vi "Fetch2ChSegHZOffset.vi"(9 "2nd Channel?":bool, 10 "Num Segs":i32=50, 11 "VISA resource name":refnum<visa-resource-name>="HDO6104") -> (0 "Run Time":u32, 1 "Array 2":dbl[](array[numeric]), 2 "Array":dbl[](array[numeric]), 3 "VISA resource name out":refnum<visa-resource-name>)   [LabVIEW 2022 SP3]
uses:
  <instrlib>/LeCroy Wave Series/LeCroy Wave Series.lvlib
panel:
  out "CH2 HZ Offset":dbl[](graph)
  out "CH1 HZ Offset":dbl[](graph)
  out "x-y":dbl[](array[numeric])
  out "Offset differences":dbl[](graph)
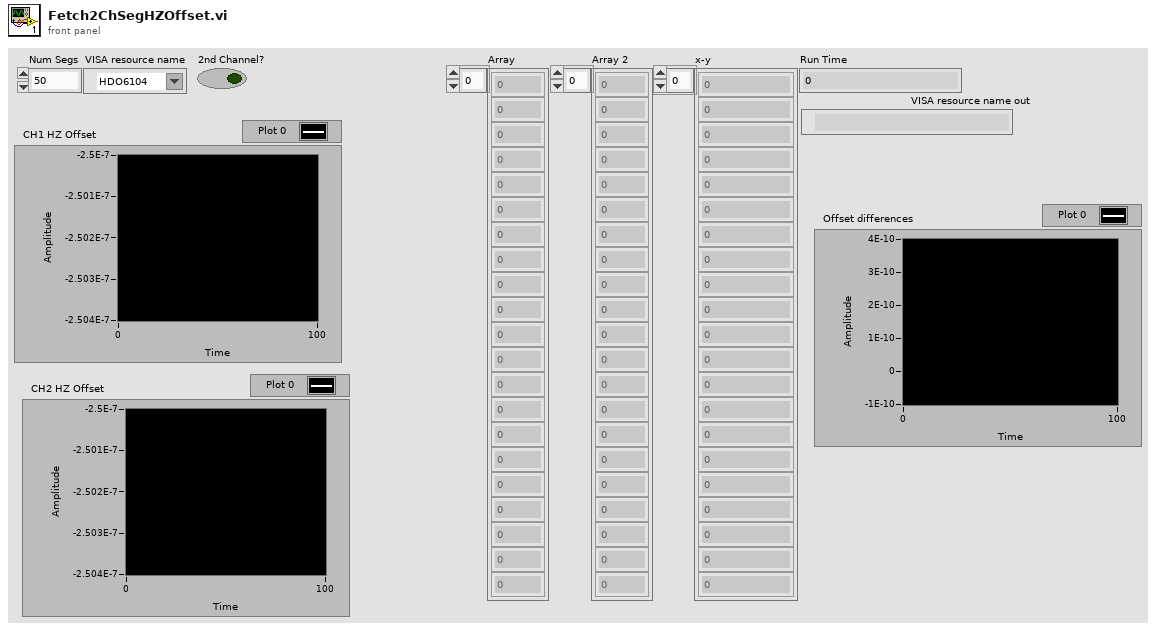
[diagram p1: front panel]
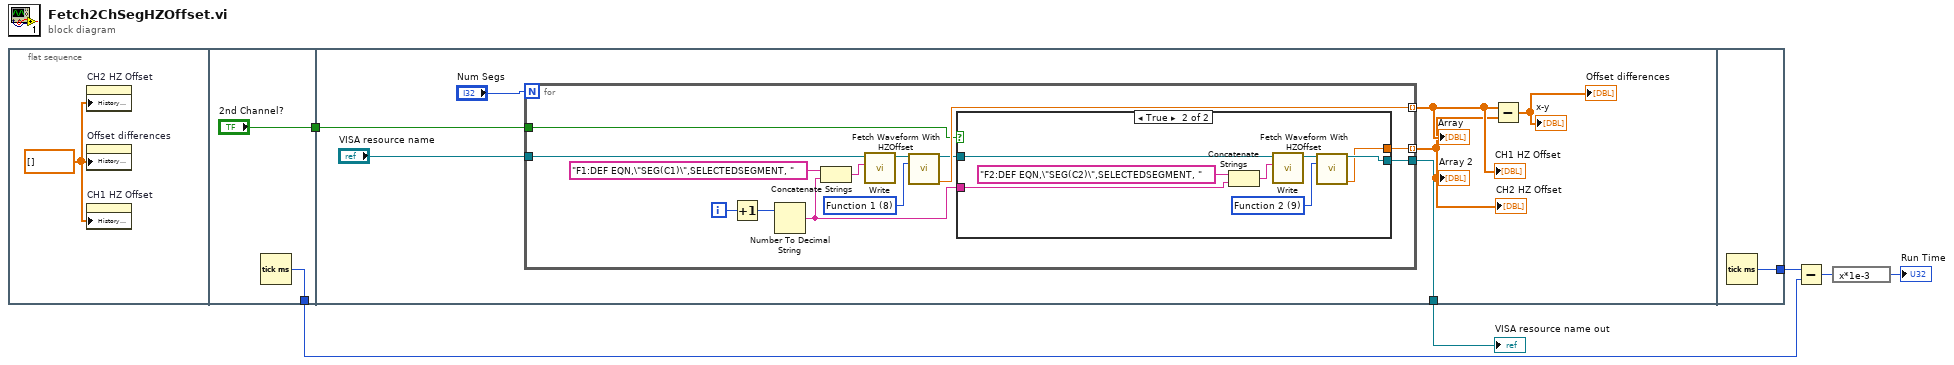
[diagram p0: block diagram]
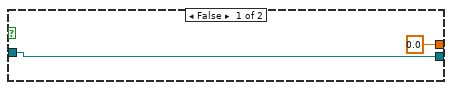
[diagram p2: hidden frame]
diagram:
  n1 = flat-sequence {
    tunnel: [w9] -> w3
    tunnel: ["2nd Channel?"] -> w1
    tunnel: [w12] -> w2
    tunnel: w1 -> [w11]
    tunnel: [w40] -> w4
    frame #0 {
      w7 = dbl[] [] ("History Data")
      n2 = property on="CH2 HZ Offset" class="WFChart (strict)"("History Data"=w7) -> ()  [unwired: 2 in, 2 out]
      n3 = property on="Offset differences" class="WFChart (strict)"("History Data"=w7) -> ()  [unwired: 2 in, 2 out]
      n4 = property on="CH1 HZ Offset" class="WFChart (strict)"("History Data"=w7) -> ()  [unwired: 2 in, 2 out]
    }
    frame #1 {
      n5 = Tick Count (ms)() -> (millisecond timer value=w9:u32)
    }
    frame #2 {
      n6 = for {
        N: "Num Segs" -> [_]
        tunnel: "VISA resource name" -> [w25]
        tunnel: [w28] -> w13 mode=indexing
        tunnel: [w20] -> w12
        tunnel: w11 -> [w18]
        tunnel: [w17] -> w10 mode=indexing
        i -> [w23]
        w29 = u16 8 items=["Channel 1", "Channel 2", "Channel 3", "Channel 4", "Memory 1", "Memory 2", "Memory 3", "Memory 4", "Function 1", "Function 2", "Function 3", "Function 4", "Function 5", "Function 6", "Function 7", "Function 8", "Other"] ("Source (0: Channel 1)")
        n7 = Increment(x=w23) -> (x+1=w22:i32)
        n8 = Number To Decimal String(number=w22) -> (decimal integer string=w21:string)  [unwired: 1 in]
        n9 = Concatenate Strings("F1:DEF EQN,\"SEG(C1)\",SELECTEDSEGMENT, " ("Write Buffer"), w21) -> (w24:string)
        n10 = call <instrlib>:"Write.vi"("Write Buffer"=w24, "VISA resource name"=w25) -> ("VISA resource name out"=w26:refnum<visa-resource-name>)  [unwired: 7 in, 2 out]
        n11 = call "Fetch Waveform With HZOffset.vi"("VISA resource name"=w26, "Source (0: Channel 1)"=w29) -> ("VISA resource name out"=w19:refnum<visa-resource-name>, "Horizontal Offset"=w28:dbl)  [unwired: 10 in, 2 out]
        n12 = case shown="True" w18 {
          tunnel: w21 -> [_ w38]
          tunnel: [w31 w37] -> w20
          tunnel: w19 -> [w31 w33]
          tunnel: [0.0 ("Horizontal Offset") w32] -> w17
          frame False {
          }
          frame True {
            w34 = u16 9 items=["Channel 1", "Channel 2", "Channel 3", "Channel 4", "Memory 1", "Memory 2", "Memory 3", "Memory 4", "Function 1", "Function 2", "Function 3", "Function 4", "Function 5", "Function 6", "Function 7", "Function 8", "Other"] ("Source (0: Channel 1)")
            n13 = Concatenate Strings("F2:DEF EQN,\"SEG(C2)\",SELECTEDSEGMENT, " ("Write Buffer"), w38) -> (w36:string)
            n14 = call <instrlib>:"Write.vi"("Write Buffer"=w36, "VISA resource name"=w33) -> ("VISA resource name out"=w35:refnum<visa-resource-name>)  [unwired: 7 in, 2 out]
            n15 = call "Fetch Waveform With HZOffset.vi"("VISA resource name"=w35, "Source (0: Channel 1)"=w34) -> ("VISA resource name out"=w37:refnum<visa-resource-name>, "Horizontal Offset"=w32:dbl)  [unwired: 10 in, 2 out]
          }
        }
      }
      "Array" <- w13
      "Array 2" <- w10
      "CH1 HZ Offset" <- w13
      "CH2 HZ Offset" <- w10
      n16 = Subtract(x=w13, y=w10) -> (x-y=→"Offset differences" →"x-y":dbl[])
    }
    frame #3 {
      n17 = Tick Count (ms)() -> (millisecond timer value=w40:u32)
    }
  }
  n18 = Subtract(x=w4, y=w3) -> (x-y=w6:u32)
  n19 = expression code="x*1e-3"(w6) -> (→"Run Time":u32)
  "VISA resource name out" <- w2
